vi "readSMGR.vi"(4 "error in":errorcluster, 7 "file path":path) -> (0 "error out":errorcluster, 1 "output array":waveform(i16)[][](array[waveform]), 2 "sync":waveform(i16)(graph))   [LabVIEW 2010]
panel:
  out "relative t":dbl format="%#_6p"
  out "element":timestamp format="%<%.7X\n%x>T"
  in  "piece":i32 min=0 max=42
  out "SMGR":string
  out "pieces":i32
  out "Waveform Graph":waveform(i16)[](graph)
  out "meas_point":string
  out "max_value":i16
  out "Table":string[][](table)
  out "path":path
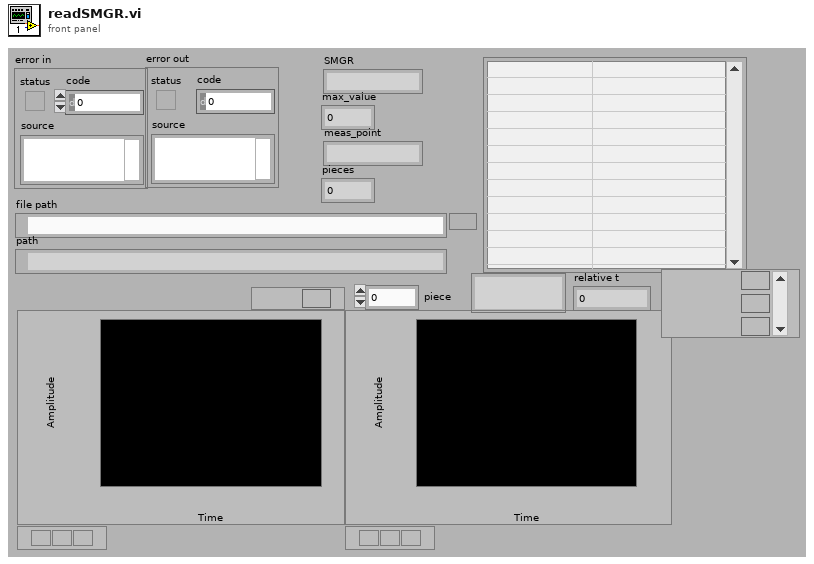
[diagram p1: front panel]
types:
  T1 = typedef "LVDateTimeRec.ctl" = cluster{"fractional second":dbl, "second":i32, "minute":i32, "hour":i32, "day of month":i32, "month":i32, "year":i32, "day of week":i32, "day of year":i32, "DST":i32}
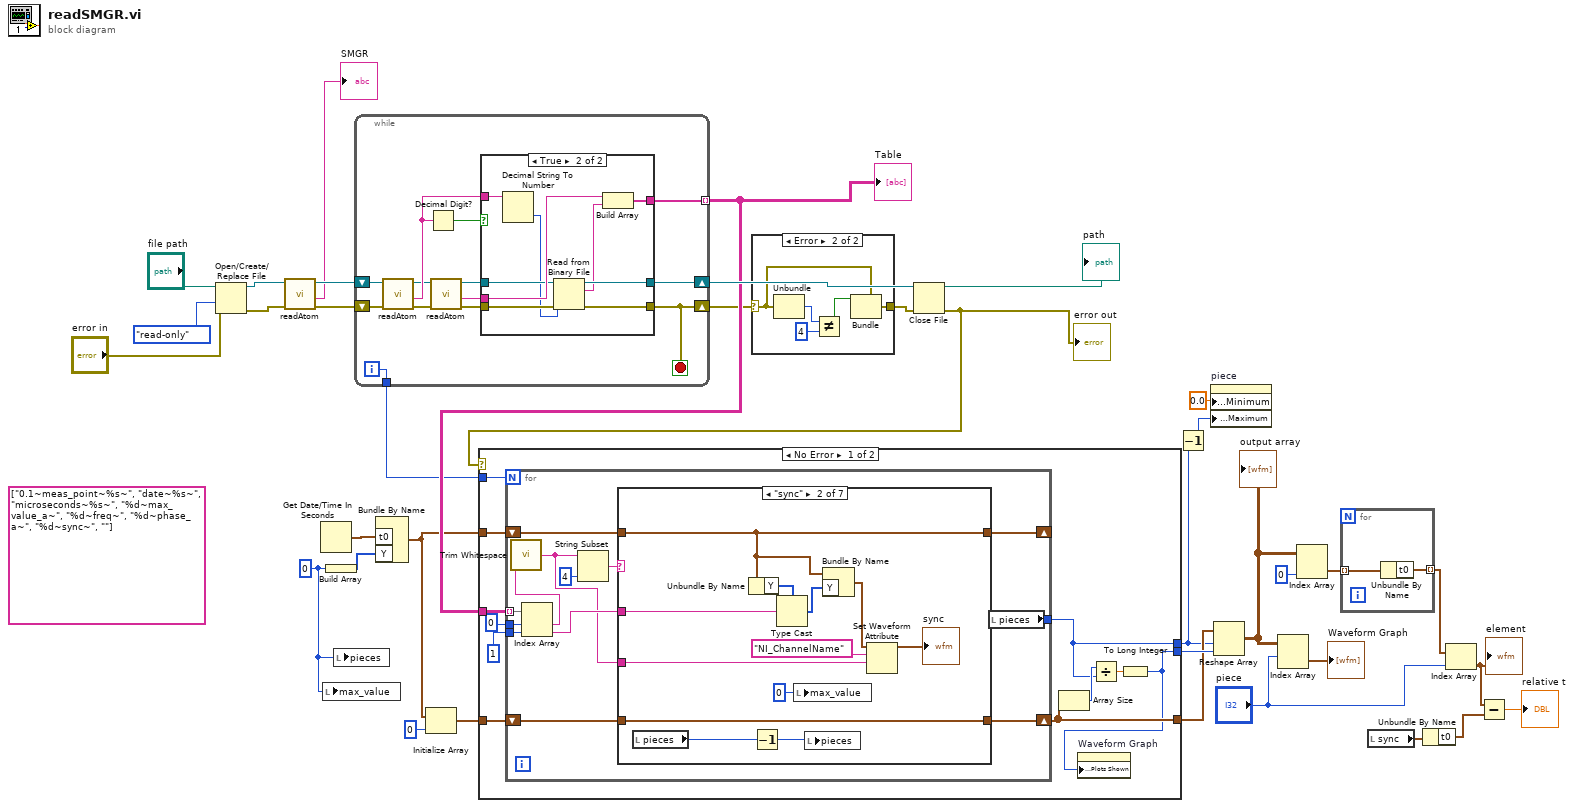
[diagram p0: block diagram]
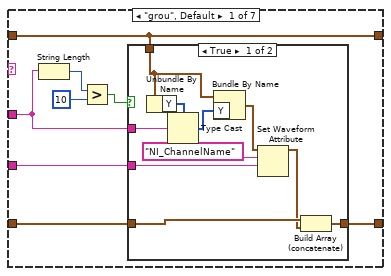
[diagram p2: hidden frame]
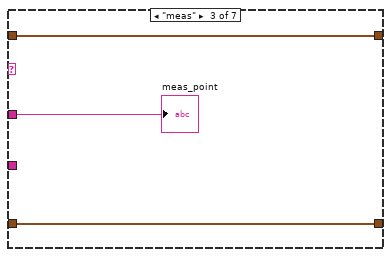
[diagram p4: hidden frame]
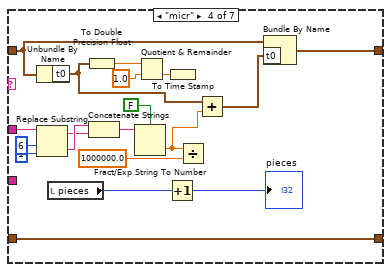
[diagram p5: hidden frame]
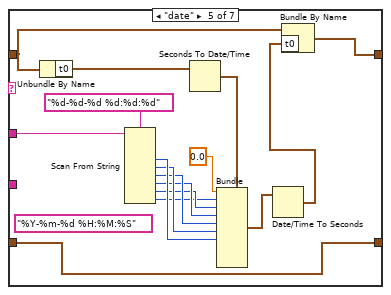
[diagram p6: hidden frame]
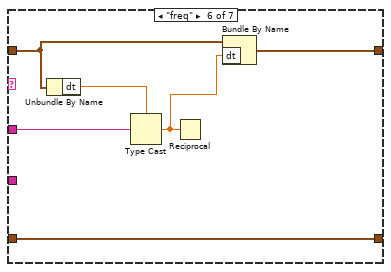
[diagram p7: hidden frame]
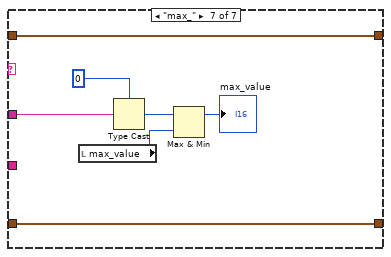
[diagram p8: hidden frame]
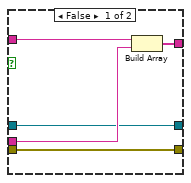
[diagram p11: hidden frame]
diagram:
  (unwired) string[] ["0.1~meas_point~%s~", "date~%s~", "microseconds~%s~", "%d~max_value_a~", "%d~freq~", "%d~phase_a~", "%d~sync~", ""]
  w1 = i16 0
  n1 = Open/Create/Replace File(file path (use dialog)="file path", error in="error in", access (0:read/write)=enum16{"read/write", "read-only", "write-only"}."read-only") -> (refnum out=w32:refnum<file>, error out=w31:errorcluster)  [unwired: 3 in, 1 out]
  n2 = call "readAtom.vi"("error in"=w31, "Byte Stream File"=w32) -> ("error out"=w29:errorcluster, "String"=→"SMGR":string, "Byte Stream File Refnum"=w30:refnum<file>)  [unwired: 3 in]
  n3 = Get Date/Time In Seconds() -> (seconds since 1Jan1904=w26:timestamp)
  n4 = local write "max_value"(w1) -> ()
  n5 = Build Array(w1) -> (w25:i16[])
  n6 = local write "pieces"(w1) -> ()
  n7 = while {
    shift-right: [w39] -> w20
    shift-left: w29 -> [w49]
    shift-right: [w40] -> w33
    shift-left: w30 -> [w48]
    tunnel: [w45] -> w27 mode=indexing
    tunnel: [w37] -> w21
    i -> [w37]
    stop <- w39 stop-if-true
    n8 = call "readAtom.vi"("error in"=w49, "Byte Stream File"=w48) -> ("error out"=w43:errorcluster, "String"=w46:string, "Byte Stream File Refnum"=w44:refnum<file>)  [unwired: 3 in]
    n9 = Decimal Digit?(1:w46) -> (0:w47:bool)
    n10 = call "readAtom.vi"("error in"=w43, "Byte Stream File"=w44) -> ("error out"=w38:errorcluster, "String"=w41:string, "Byte Stream File Refnum"=w42:refnum<file>)  [unwired: 3 in]
    n11 = case shown="True" w47 {
      tunnel: w42 -> [w51 w62]
      tunnel: w38 -> [w50 w61]
      tunnel: w46 -> [w54 w57]
      tunnel: [w53 w60] -> w45
      tunnel: w41 -> [w52 w63]
      tunnel: [w51 w59] -> w40
      tunnel: [w50 w58] -> w39
      frame False {
        n12 = Build Array(w54, w52) -> (w53:string[])
      }
      frame True {
        n13 = Decimal String To Number(string=w57) -> (number=w56:i32)  [unwired: 2 in, 1 out]
        n14 = Read from Binary File(8:w61, 10:w56, 11:w62) -> (0:w58:errorcluster, 2:w55:string, 3:w59:refnum<file>)  [unwired: 3 in, 1 out]
        n15 = Build Array(w63, w55) -> (w60:string[])
      }
    }
  }
  "Table" <- w27
  n16 = Bundle By Name("t0"=w26, "Y"=w25) -> (w23:waveform(i16))  [unwired: 1 in]
  n17 = Initialize Array(w23, 0 ("dimension size")) -> (w22:waveform(i16)[])
  n18 = case shown="Error" w20 {
    selector: w20 -> [w64 w67]
    tunnel: [w64 w65] -> w19
    frame No Error {
    }
    frame Error {
      n19 = Unbundle(w67) -> ("code"=w69:i32)  [unwired: 2 out]
      n20 = Not Equal?(x=w69, y=4) -> (x != y?=w66:bool)
      n21 = Bundle(cluster=w67, "status"=w66) -> (w65:errorcluster)  [unwired: 2 in]
    }
  }
  n22 = Close File(refnum=w33, error in=w19) -> (path=→"path":path, error out=w18:errorcluster)
  "error out" <- w18
  n23 = case shown="No Error" w18 {
    tunnel: w27 -> [w80 _]
    tunnel: w23 -> [w77 _]
    tunnel: w22 -> [w76 w176]
    tunnel: [w73 w176] -> w16
    tunnel: w21 -> [w75 _]
    tunnel: [w70 _] -> w13
    tunnel: [w71 _] -> w17
    frame No Error {
      n24 = for {
        N: w75 -> [_]
        tunnel: w80 -> [w93] mode=indexing
        tunnel: 0 -> [w92]
        tunnel: 1 -> [w91]
        shift-right: [w89] -> _
        shift-left: w77 -> [w90]
        shift-right: [w86] -> w73
        shift-left: w76 -> [w87]
        tunnel: [w85] -> w70
        n25 = Index Array(array=w93, index #1=w92, index #2=w91) -> (element #1=w82:string, element #2=w88:string)
        n26 = call <vilib>:"Trim Whitespace.vi"("string"=w82) -> ("trimmed string"=w81:string)  [unwired: 1 in]
        n27 = String Subset(string=w81, length (rest)=4 ("length (rest)")) -> (substring=w84:string)  [unwired: 1 in]
        n28 = case shown="\"sync\"" w84 {
          tunnel: w90 -> [w95 w124 w125 w145 w160 w167 w172]
          tunnel: [w95 w124 w125 w141 w158 w163 w172] -> w89
          tunnel: w88 -> [w99 w123 w126 w133 w161 w168 w174]
          tunnel: w87 -> [w101 w122 w127 w143 w159 w165 w175]
          tunnel: [w100 w122 w127 w143 w159 w165 w175] -> w86
          tunnel: w81 -> [w94 w114 _ _ _ _ _]
          frame "grou", Default {
            n29 = String Length(string=w99) -> (length=w98:i32)
            n30 = Greater?(x=w98, y=10) -> (0:w96:bool)
            n31 = case shown="True" w96 {
              tunnel: w101 -> [w111 w112]
              tunnel: [w110 w112] -> w100
              tunnel: w99 -> [w109 _]
              tunnel: w95 -> [w108 _]
              tunnel: w94 -> [w103 _]
              frame True {
                n32 = Unbundle By Name(w108) -> ("Y"=w107:i16[])
                n33 = Type Cast(type=w107, x=w109) -> (*(type *) &x=w106:i16[])
                n34 = Bundle By Name(cluster=w108, "Y"=w106) -> (w105:waveform(i16))
                n35 = Set Waveform Attribute(5:w103, 6:"NI_ChannelName" ("name"), 7:w105) -> (3:w104:waveform(i16))  [unwired: 1 in, 2 out]
                n36 = Build Array (concatenate)(w111, w104) -> (w110:waveform(i16)[])
              }
              frame False {
              }
            }
          }
          frame "sync" {
            n37 = local read "pieces"() -> (w121:i32)
            n38 = Unbundle By Name(w124) -> ("Y"=w119:i16[])
            n39 = Decrement(x=w121) -> (x-1=w120:i32)
            n40 = Type Cast(type=w119, x=w123) -> (*(type *) &x=w118:i16[])
            n41 = local write "max_value"(i16 0 ("max_value")) -> ()
            n42 = local write "pieces"(w120) -> ()
            n43 = Bundle By Name(cluster=w124, "Y"=w118) -> (w117:waveform(i16))
            n44 = Set Waveform Attribute(5:w114, 6:"NI_ChannelName" ("name"), 7:w117) -> (3:→"sync":waveform(i16))  [unwired: 1 in, 2 out]
          }
          frame "meas" {
            "meas_point" <- w126
          }
          frame "micr" {
            n45 = Unbundle By Name(w145) -> ("t0"=w128:timestamp)
            n46 = Replace Substring(2:1 ("length (len. of substring)"), 3:6 ("offset (0)"), 5:w133) -> (0:w135:string, 1:w134:string)  [unwired: 1 in]
            n47 = local read "pieces"() -> (w142:i32)
            n48 = To Double Precision Float(number=w128) -> (double precision float=w140:dbl)
            n49 = Concatenate Strings(w135, w134) -> (w132:string)
            n50 = Fract/Exp String To Number(use system decimal point (T)=FALSE, string=w132) -> (number=w129:dbl)  [unwired: 2 in, 1 out]
            n51 = Quotient & Remainder(x=w140, y=1.0) -> (floor(x/y)=w138:dbl)  [unwired: 1 out]
            n52 = Increment(x=w142) -> (x+1=→"pieces":i32)
            n53 = To Time Stamp(1:w138) -> ()  [unwired: 1 out]
            n54 = Divide(x=w129, y=1000000.0) -> ()  [unwired: 1 out]
            n55 = Add(x=w128, y=w129) -> (x+y=w144:timestamp)
            n56 = Bundle By Name(cluster=w145, "t0"=w144) -> (w141:waveform(i16))
          }
          frame "date" {
            (unwired) "%Y-%m-%d %H:%M:%S" ("time format string (%c)")
            n57 = Unbundle By Name(w160) -> ("t0"=w157:timestamp)
            n58 = Scan From String(format string="%d-%d-%d %d:%d:%d", input string=w161) -> (output 1=w153:i32, output 2=w152:i32, output 3=w151:i32, output 4=w150:i32, output 5=w149:i32, output 6=w148:i32)  [unwired: 8 in, 3 out]
            n59 = Seconds To Date/Time(time stamp (now)=w157) -> (date time rec=w156:T1)  [unwired: 1 in]
            n60 = Bundle(cluster=w156, "fractional second"=0.0, "second"=w148, "minute"=w149, "hour"=w150, "day of month"=w151, "month"=w152, "year"=w153) -> (w155:T1)  [unwired: 3 in]
            n61 = Date/Time To Seconds(2:w155) -> (0:w154:timestamp)  [unwired: 1 in]
            n62 = Bundle By Name(cluster=w160, "t0"=w154) -> (w158:waveform(i16))
          }
          frame "freq" {
            n63 = Unbundle By Name(w167) -> ("dt"=w166:dbl)
            n64 = Type Cast(type=w166, x=w168) -> (*(type *) &x=w164:dbl)
            n65 = Reciprocal(x=w164) -> ()  [unwired: 1 out]
            n66 = Bundle By Name(cluster=w167, "dt"=w164) -> (w163:waveform(i16))
          }
          frame "max_" {
            n67 = local read "max_value"() -> (w170:i16)
            n68 = Type Cast(type=i16 0 ("max_value"), x=w174) -> (*(type *) &x=w171:i16)
            n69 = Max & Min(x=w171, y=w170) -> (max(x,y)=→"max_value":i16)  [unwired: 1 out]
          }
        }
        n70 = local read "pieces"() -> (w85:i32)
      }
      n71 = Array Size(array=w73) -> (size(s)=w74:i32)
      n72 = Divide(x=w74, y=w70) -> (x/y=w72:dbl)
      n73 = To Long Integer(number=w72) -> (32bit integer=w71:i32)
      n74 = property on="Waveform Graph" class="WFGraph (strict)"("Legend:Plots Shown"=w71) -> ()  [unwired: 2 in, 2 out]
    }
    frame Error {
    }
  }
  n75 = Decrement(x=w13) -> (x-1=w12:i32)
  n76 = property on="piece" class="DigNum (strict)"("Data Entry Limits:Minimum"=0.0 ("Data Range:Minimum"), "Data Entry Limits:Maximum"=w12) -> ()  [unwired: 2 in, 2 out]
  n77 = Reshape Array(w16, w13, w17) -> (w10:waveform(i16)[][])
  "output array" <- w10
  n78 = Index Array(array=w10, index (row)="piece") -> (element=→"Waveform Graph":waveform(i16)[])  [unwired: 1 in]
  n79 = Index Array(array=w10, index (col)=0) -> (element=w9:waveform(i16)[])  [unwired: 1 in]
  n80 = for {
    tunnel: w9 -> [w178] mode=indexing
    tunnel: [w177] -> w7 mode=indexing
    n81 = Unbundle By Name(w178) -> ("t0"=w177:timestamp)
  }
  n82 = local read "sync"() -> (w6:waveform(i16))
  n83 = Unbundle By Name(w6) -> ("t0"=w4:timestamp)
  n84 = Index Array(array=w7, index="piece") -> (element=w5:timestamp)
  "element" <- w5
  n85 = Subtract(x=w5, y=w4) -> (x-y=→"relative t":dbl)
